vi "Sort Population In Descending Order.vi"(11 "Population":T1[](array[typedef])) -> (2 "Population In Descending Order":T1[](array[typedef]), 3 "Fitness Values In Descending Order":u16[](array[numeric]))   [LabVIEW 2013, in "GA.lvclass"]
uses:
  GA.lvclass
  Controls/Solution_GA.ctl
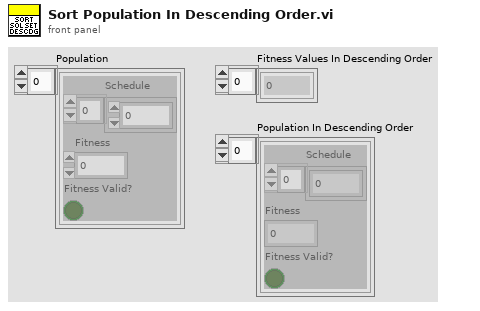
[diagram p1: front panel]
types:
  T1 = typedef "Solution_GA.ctl" = cluster{"Schedule":u16[], "Fitness":u16, "Fitness Valid?":bool}
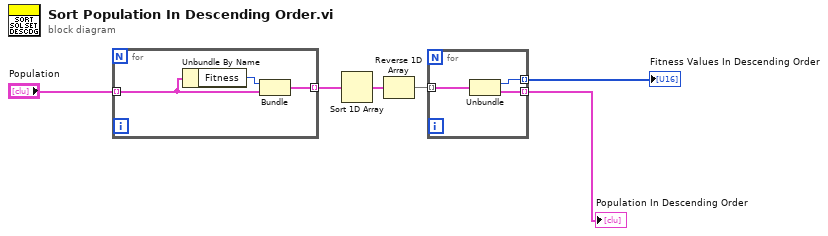
[diagram p0: block diagram]
diagram:
  n1 = for {
    tunnel: [w9] -> w3 mode=indexing
    tunnel: "Population" -> [w8] mode=indexing
    n2 = Unbundle By Name(w8) -> ("Fitness"=w7:u16)
    n3 = Bundle("Fitness"=w7, "Solution"=w8) -> (w9:cluster{"Fitness":u16, "Solution":T1})  [unwired: 1 in]
  }
  n4 = Sort 1D Array(array=w3) -> (sorted array=w2:cluster{"Fitness":u16, "Solution":T1}[])
  n5 = Reverse 1D Array(array=w2) -> (reversed array=w1:cluster{"Fitness":u16, "Solution":T1}[])
  n6 = for {
    tunnel: [w12] -> w6 mode=indexing
    tunnel: [w11] -> w5 mode=indexing
    tunnel: w1 -> [w10] mode=indexing
    n7 = Unbundle(w10) -> ("Fitness"=w11:u16, "Solution"=w12:T1)
  }
  "Population In Descending Order" <- w6
  "Fitness Values In Descending Order" <- w5
